vi "Test TCC Request Chamber State Returns Setpoint.vi"(8 "error in (no error)":errorcluster, 11 "Thermal Chamber Controller Test In":refnum<class "Thermal Chamber Controller Test.lvclass">) -> (0 "error out":errorcluster, 3 "Thermal Chamber Controller Test Out":refnum<class "Thermal Chamber Controller Test.lvclass">)   [LabVIEW 2020, in "Thermal Chamber Controller Test.lvclass"]
uses:
  Thermal Chamber Controller Test.lvclass
  C:/Program Files (x86)/National Instruments/LabVIEW 2020/vi.lib/Astemes/LUnit/Test Case.lvclass
  Thermal Chamber Controller/Thermal Chamber Controller.lvclass
  C:/Program Files (x86)/National Instruments/LabVIEW 2020/vi.lib/Astemes/Triarc Framework/Process/Process.lvclass
  <vilib>/Astemes/Triarc Framework/Process/Process.lvclass/Process.ctl
  <vilib>/Astemes/LUnit/Test Case.lvclass/Test Case.ctl
  dc438c5f-6843-4ac9-a0a6-ca91c263d498.vi
  <vilib>/Astemes/Triarc Framework/Process/Private/SubVIs/Wait for finish.vi
  <vilib>/Astemes/Triarc Framework/Process/Private/SubVIs/Set Lifecycle State.vi
  <vilib>/Astemes/Triarc Framework/Process/Protected/Messaging/Send Message.vi
  <vilib>/Astemes/LUnit/Core/LUnit Test Case/Private/Append Pass Result.vi
  <vilib>/Astemes/LUnit/Core/LUnit Test Case/Private/Append Fail Result.vi
  dc438c5f-6843-4ac9-a0a6-ca91c263d498.vi/9c5d11cd-9439-4240-a1ee-d9baace9c924.vi
  <vilib>/Astemes/Triarc Framework/Process/Private/SubVIs/Handle Debug Data.vi
  <vilib>/Astemes/LUnit/Core/LUnit Test Case/Private/Run In UI.vi
  <vilib>/Utility/error.llb/Clear Errors.vi
  <vilib>/Astemes/Triarc Framework/Process/Public/Lifecycle/Get Lifecycle State.vi
  <vilib>/Utility/error.llb/Error Cluster From Error Code.vi
  <vilib>/Astemes/Triarc Framework/Callback/Callback.lvclass
  <vilib>/Astemes/Triarc Framework/Process/Process.lvclass
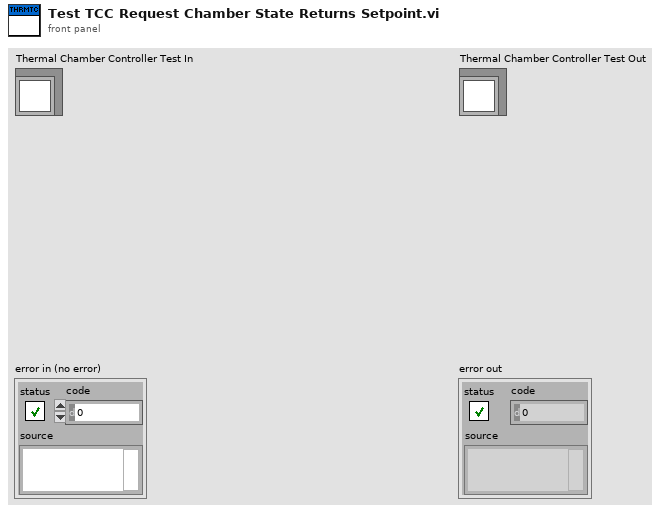
[diagram p1: front panel]
types:
  T1 = typedef "Thermal Chamber Controller.lvclass/Chamber State.ctl" = cluster{"Actual Temperature":dbl, "Temperature Set Point":dbl, "Temperature Ramp Rate":dbl, "Heater State":T2}
  T2 = typedef "Thermal Chamber Controller.lvclass/Heater State.ctl" = enum16{"Heater Disabled", "Heater Enabled"}
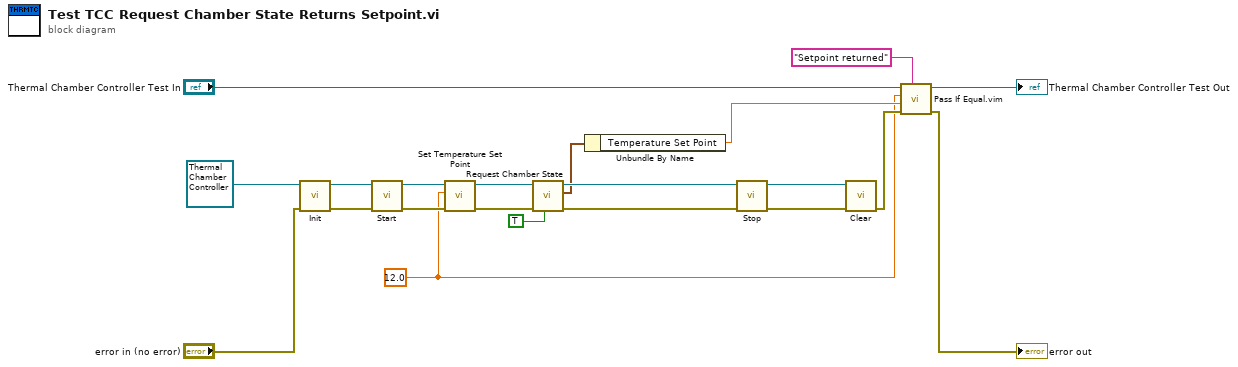
[diagram p0: block diagram]
diagram:
  w1 = 12.0 ("Temperature Set Point")
  n1 = call-dynamic "Init.vi"("error in (no error)"="error in (no error)", "View In"=refnum<class "Thermal Chamber Controller.lvclass"> refnum ("Thermal Chamber Controller.lvclass")) -> ("error out"=w15:errorcluster, "View Out"=w16:refnum<class "Thermal Chamber Controller.lvclass">)  [unwired: 8 in]
  n2 = call <vilib>:"Start.vi"("error in (no error)"=w15, "Process In"=w16) -> ("error out"=w20:errorcluster, "Process Out"=w7:refnum<class "Thermal Chamber Controller.lvclass">)  [unwired: 7 in, 1 out]
  n3 = call "Set Temperature Set Point.vi"("error in (no error)"=w20, "Temperature Set Point"=w1, "Thermal Chamber Controller In"=w7) -> ("error out"=w9:errorcluster, "Thermal Chamber Controller Out"=w8:refnum<class "Thermal Chamber Controller.lvclass">)  [unwired: 7 in]
  n4 = call "Request Chamber State.vi"("wait for reply (T)"=TRUE, "error in (no error)"=w9, "Thermal Chamber Controller In"=w8) -> ("error out"=w14:errorcluster, "Chamber Status Reply Payload"=w10:T1, "Thermal Chamber Controller Out"=w19:refnum<class "Thermal Chamber Controller.lvclass">)  [unwired: 5 in, 1 out]
  n5 = Unbundle By Name(w10) -> ("Temperature Set Point"=w2:dbl)
  n6 = call <vilib>:"Stop.vi"("error in (no error)"=w14, "Process In"=w19) -> ("error out"=w17:errorcluster, "Process Out"=w18:refnum<class "Thermal Chamber Controller.lvclass">)  [unwired: 7 in, 1 out]
  n7 = call-dynamic "Clear.vi"("error in (no error)"=w17, "View In"=w18) -> ("error out"=w5:errorcluster)  [unwired: 9 in]
  n8 = call "Pass If Equal.vim"("Description"="Setpoint returned", "error in (no error)"=w5, "Actual"=w2, "Expected"=w1, "LUnit Test Case In"="Thermal Chamber Controller Test In") -> ("error out"=→"error out":errorcluster, "LUnit Test Case Out"=→"Thermal Chamber Controller Test Out":refnum<class "Thermal Chamber Controller Test.lvclass">)  [unwired: 5 in]
